vi "Get Child Tag.vi"(10 "Child label":string, 11 "Parent tag":string) -> (3 "Child tag":string)   [LabVIEW 2020, in "Output Sequencer.lvlib" / "Settings UI.lvclass"]
uses:
  Settings UI.lvclass
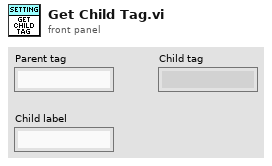
[diagram p1: front panel]
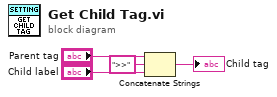
[diagram p0: block diagram]
diagram:
  n1 = Concatenate Strings("Parent tag", ">>" ("string"), "Child label") -> (→"Child tag":string)
